vi "Washing_Process (SubVI).vi"(10 "Array in":string[](array[string]), 11 "Digital in":refnum<vi>) -> (1 "Boolean":bool, 2 "Array out":string[](array[string]), 3 "empty?":bool)   [LabVIEW 2019]
uses:
  a44d899a-b465-4466-b89f-fb14948e60c4.vi
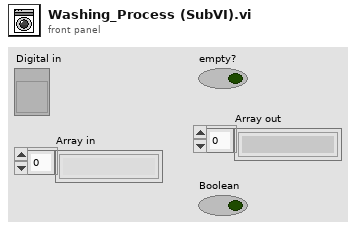
[diagram p1: front panel]
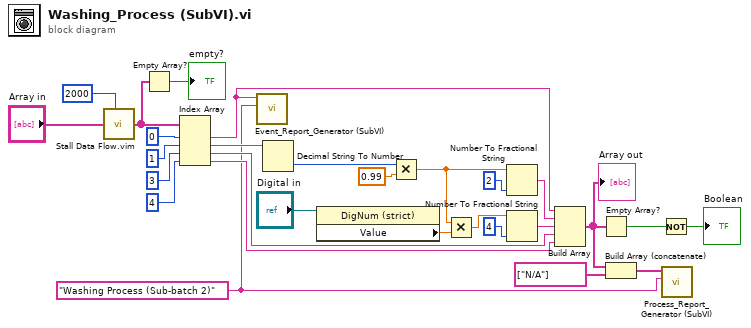
[diagram p0: block diagram]
diagram:
  w4 = "Washing Process (Sub-batch 2)" ("Process Name")
  n1 = call "Stall Data Flow.vim"("value in"="Array in", "milliseconds to wait"=u32 2000) -> ("value out"=w13:string[])  [unwired: 1 out]
  n2 = Empty Array?(array=w13) -> (empty?=→"empty?":bool)
  n3 = Index Array(array=w13, index #1=0 ("index"), index #2=1 ("index"), index #3=3 ("index"), index #4=4 ("index")) -> (element #1=w5:string, element #2=w21:string, element #3=w25:string, element #4=w26:string)
  n4 = call "Event_Report_Generator (SubVI).vi"("Process Name"=w4, "Booking ID"=w5) -> ()  [unwired: 10 in]
  n5 = Decimal String To Number(string=w21) -> (number=w28:i32)  [unwired: 2 in, 1 out]
  n6 = property class="DigNum (strict)"(reference="Digital in") -> ("Value"=w20:dbl)  [unwired: 1 in, 2 out]
  n7 = Multiply(x=w28, y=0.99) -> (x*y=w17:dbl)
  n8 = Multiply(x=w17, y=w20) -> (x*y=w19:dbl)
  n9 = Number To Fractional String(number=w17, precision (6)=i16 2) -> (F-format string=w23:string)  [unwired: 2 in]
  n10 = Number To Fractional String(number=w19, precision (6)=i16 4) -> (F-format string=w24:string)  [unwired: 2 in]
  n11 = Build Array(w5, w23, w24, w25, w26) -> (w3:string[])
  "Array out" <- w3
  n12 = Empty Array?(array=w3) -> (empty?=w15:bool)
  n13 = Build Array (concatenate)(w3, string[] ["N/A"] ("array")) -> (w1:string[])
  n14 = Not(x=w15) -> (.not. x?=→"Boolean":bool)
  n15 = call "Process_Report_Generator (SubVI).vi"("Process Name"=w4, "Process Information"=w1) -> ()  [unwired: 10 in]
